vi "set_scattering_length.vi"(8 "error in (no error)":errorcluster, 10 "scattering length":dbl[unit], 11 "GenericTrajectory.lvclass in":refnum<class "TrajectoryDL091126GenericVoxel.lvclass">) -> (0 "error out":errorcluster, 3 "GenericTrajectory.lvclass out":refnum<class "TrajectoryDL091126GenericVoxel.lvclass">)   [LabVIEW 2010, in "TrajectoryDL091126GenericVoxel.lvclass"]
uses:
  TrajectoryDL091126GenericVoxel.lvclass
  TrajectoryDL091126GenericVoxel.lvclass/TrajectoryDL091126GenericVoxel.ctl
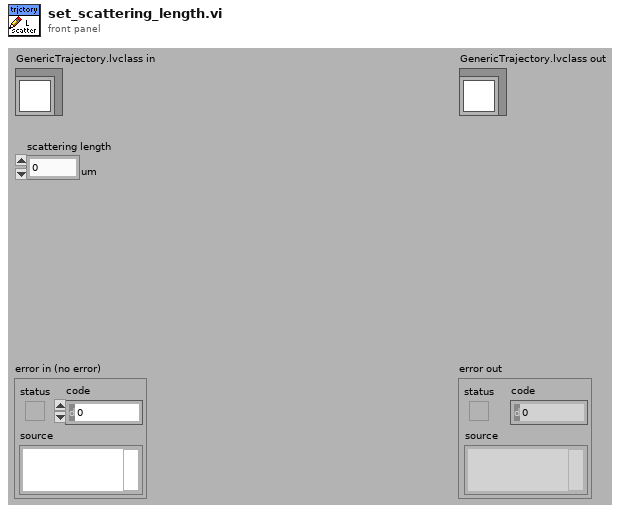
[diagram p1: front panel]
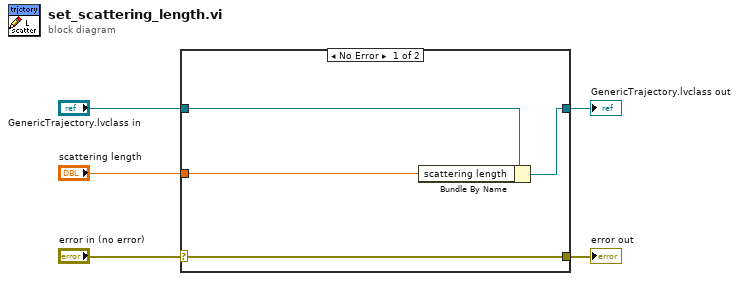
[diagram p0: block diagram]
diagram:
  n1 = case shown="No Error" "error in (no error)" {
    selector: "error in (no error)" -> [w9 w10]
    tunnel: [w9 w10] -> w4
    tunnel: [w7 w11] -> w2
    tunnel: "GenericTrajectory.lvclass in" -> [w8 w11]
    tunnel: "scattering length" -> [w6 _]
    frame No Error {
      n2 = Bundle By Name(cluster=w8, "scattering length"=w6) -> (w7:refnum<class "TrajectoryDL091126GenericVoxel.lvclass">)
    }
    frame Error {
    }
  }
  "error out" <- w4
  "GenericTrajectory.lvclass out" <- w2
